vi "Sequence Data 2d Array to Cluster.vi"(1 "data":string[][](array[string])) -> (0 "Array":T1[](array[typedef]))   [LabVIEW 2020]
uses:
  Control/Setup - Sequence Data.ctl
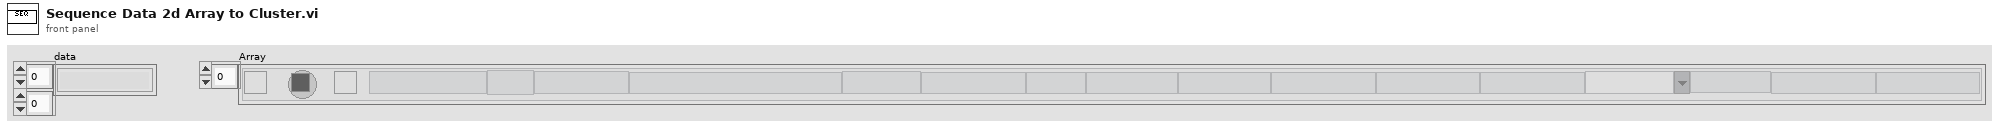
[diagram p1: front panel]
types:
  T1 = typedef "Setup - Sequence Data.ctl" = cluster{"Seq.Select":bool, "Seq.Status":u32, "Seq.Run":bool, "Seq.TestSequence":string, "Seq.No":string, "Seq.ReqID":string, "Seq.TestReq":string, "Seq.Variance":string, "Seq.TestProcedure":string, "Seq.Section":string, "Seq.TestBunker":string, "Seq.TestMedia":string, "Seq.TestPressure":string, "Seq.Cycle":string, "Seq.HoldingTime":string, "Seq.ChartScale":string, "Seq.BDIndicator":string, "Seq.ActuatorPressure":string, "Seq.MaxBDPressure":string}
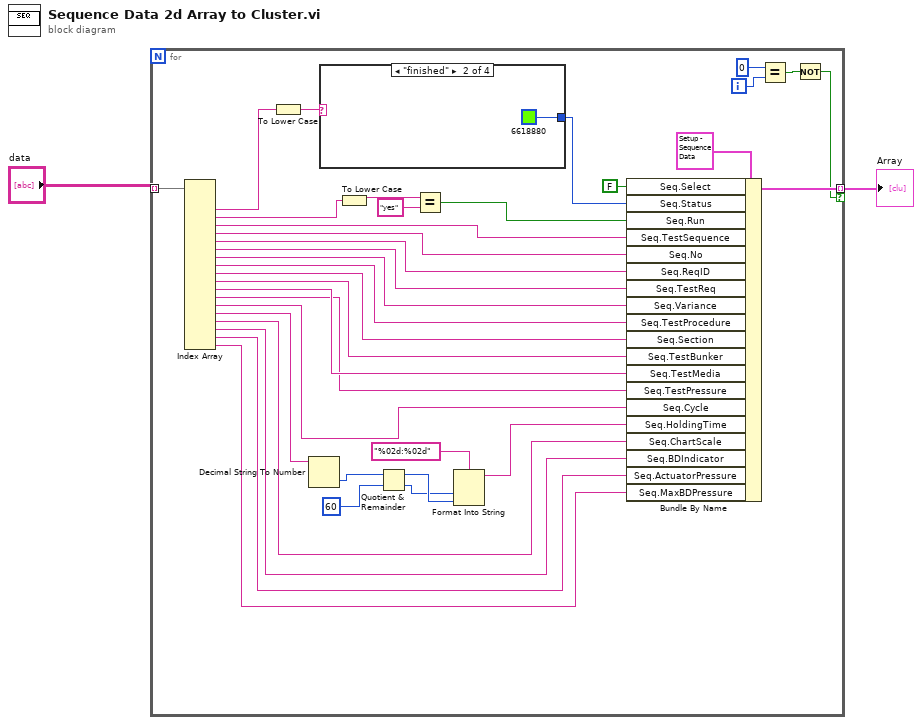
[diagram p0: block diagram]
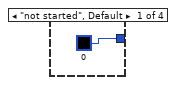
[diagram p2: hidden frame]
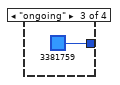
[diagram p3: hidden frame]
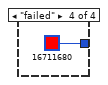
[diagram p4: hidden frame]
diagram:
  n1 = for {
    tunnel: "data" -> [w37] mode=indexing
    tunnel: [w38] -> w2 mode=indexing if=w13
    i -> [w16]
    n2 = Index Array(array=w37) -> (element #2=w4:string, element #3=w21:string, element #4=w36:string, element #5=w35:string, element #6=w34:string, element #7=w33:string, element #8=w32:string, element #9=w31:string, element #10=w30:string, element #11=w29:string, element #12=w28:string, element #13=w27:string, element #14=w26:string, element #15=w12:string, element #16=w25:string, element #17=w24:string, element #18=w23:string, element #19=w22:string)  [unwired: 19 in, 1 out]
    n3 = To Lower Case(string=w4) -> (all lower case string=w5:string)
    n4 = Decimal String To Number(string=w12) -> (number=w11:i32)  [unwired: 2 in, 1 out]
    n5 = case shown="\"finished\"" w5 {
      tunnel: [u32 0 u32 6618880 u32 3381759 u32 16711680] -> w3
      frame "not started", Default {
      }
      frame "finished" {
      }
      frame "ongoing" {
      }
      frame "failed" {
      }
    }
    n6 = To Lower Case(string=w21) -> (all lower case string=w20:string)
    n7 = Quotient & Remainder(x=w11, y=60) -> (x-y*floor(x/y)=w9:i32, floor(x/y)=w8:i32)
    n8 = Equal?(x=w20, y="yes") -> (x = y?=w18:bool)
    n9 = Format Into String(format string="%02d:%02d", w8, w9) -> (resulting string=w7:string)  [unwired: 2 in, 1 out]
    n10 = Bundle By Name(cluster=T1 {"Seq.Select"=FALSE, "Seq.Status"=0, "Seq.Run"=FALSE, "Seq.TestSequence"="", "Seq.No"="", "Seq.ReqID"="", "Seq.TestReq"="", "Seq.Variance"="", "Seq.TestProcedure"="", "Seq.Section"="", "Seq.TestBunker"="", "Seq.TestMedia"="", "Seq.TestPressure"="", "Seq.Cycle"="", "Seq.HoldingTime"="", "Seq.ChartScale"="", "Seq.BDIndicator"="", "Seq.ActuatorPressure"="", "Seq.MaxBDPressure"=""} ("Setup - Sequence Data"), "Seq.Select"=FALSE, "Seq.Status"=w3, "Seq.Run"=w18, "Seq.TestSequence"=w36, "Seq.No"=w35, "Seq.ReqID"=w34, "Seq.TestReq"=w33, "Seq.Variance"=w32, "Seq.TestProcedure"=w31, "Seq.Section"=w30, "Seq.TestBunker"=w29, "Seq.TestMedia"=w28, "Seq.TestPressure"=w27, "Seq.Cycle"=w26, "Seq.HoldingTime"=w7, "Seq.ChartScale"=w25, "Seq.BDIndicator"=w24, "Seq.ActuatorPressure"=w23, "Seq.MaxBDPressure"=w22) -> (w38:T1)
    n11 = Equal?(x=0, y=w16) -> (x = y?=w14:bool)
    n12 = Not(x=w14) -> (.not. x?=w13:bool)
  }
  "Array" <- w2
